vi "Execute.vi"(8 "error in":errorcluster, 11 "Collect Data in":refnum<class "Collect Data.lvclass">) -> (0 "error out":errorcluster, 1 "Next Step?":bool, 2 "MSG":string, 3 "Collect Data out":refnum<class "Collect Data.lvclass">)   [LabVIEW 2015, in "Collect Data.lvclass"]
uses:
  Collect Data.lvclass
  Collect Data.lvclass/Collect Data.ctl
  Reusable/Sequence/STEPS/STEP.lvclass/STEP.ctl
  Reusable/CRDS/Data/Cell/CRDS Cell Data.lvclass/CRDS Cell Data.ctl
  State data/State Data.lvclass
  State data/State Data.lvclass/State Data.ctl
  Reusable/CRDS/Data/Cell/Read extParam.vi
  State data/Write IA.vi
  State data/Write Extinction.vi
  Read # of Obs.vi
  Reusable/Sequence/STEPS/Read First Call.vi
  Read PAS DVR.vi
  Read CRD DVR.vi
  Read Associated Cells.vi
  Read Stored State DVR.vi
  Reusable/Sequence/STEPS/Write First Call.vi
  Reusable/CRDS/Data/Main/Read CellData.vi
  Reusable/Data/Read measTime.vi
  Reusable/PAS/Data/Main/Read CellData.vi
  Reusable/PAS/Data/Cell/Read derived.vi
  Data/cPAS Data.lvclass
  CRDS/Data/cCRDS Data.lvclass
  Reusable/CRDS/Data/Cell/CRDS Cell Data.lvclass
  Reusable/PAS/Data/Cell/PAS Cell Data.lvclass
  <vilib>/Analysis/NI_AALBase.lvlib
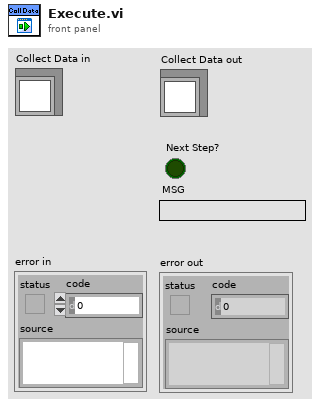
[diagram p1: front panel]
types:
  T1 = typedef "extparam.ctl" = cluster{"Tau":sgl, "Tau0cor":sgl, "ext":sgl, "extCorr":sgl, "stdevTau":sgl, "eTau":sgl, "taucorr":sgl, "Tau0":sgl, "max":sgl}
  T2 = cluster{"f0":sgl, "IA":sgl, "Q":sgl, "max":dbl[], "deltaPhi":dbl, "tau":dbl, "noiseLim":dbl, "ext":dbl}
  T3 = cluster{"Stored State":refnum<class "State Data.lvclass">[], "pointer to data":i32}
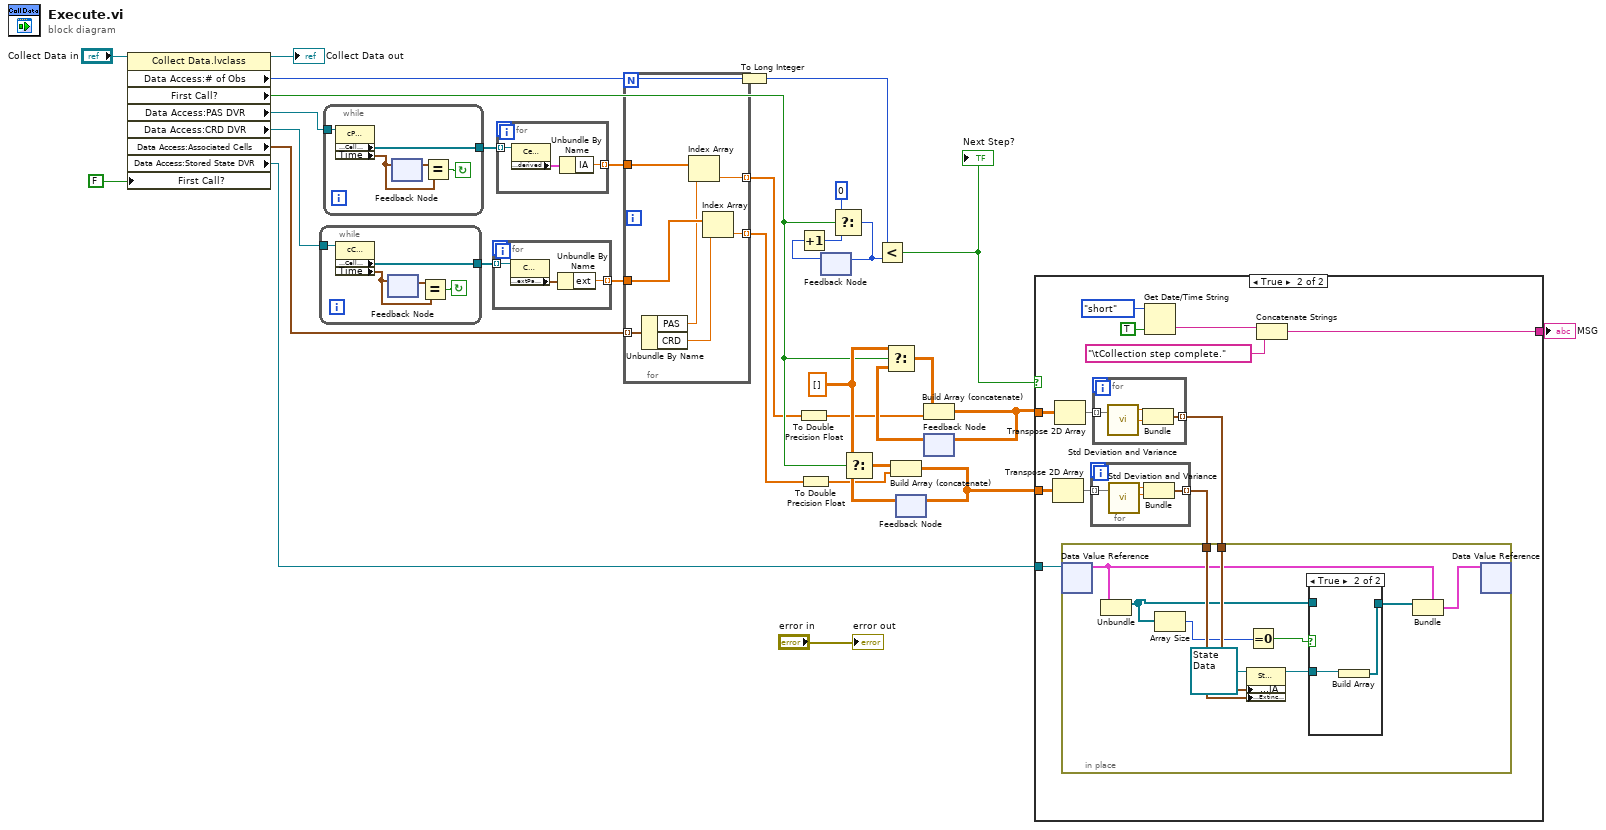
[diagram p0: block diagram]
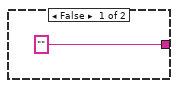
[diagram p2: hidden frame]
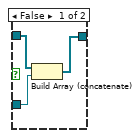
[diagram p3: hidden frame]
diagram:
  w16 = dbl[][] [] ("t")
  n1 = property class="Collect Data.lvclass"(reference="Collect Data in", "First Call?"=FALSE) -> (reference out=→"Collect Data out":refnum<class "Collect Data.lvclass">, "Data Access:# of Obs"=w6:u16, "First Call?"=w7:bool, "Data Access:PAS DVR"=w29:refnum<data-value>, "Data Access:CRD DVR"=w28:refnum<data-value>, "Data Access:Associated Cells"=w11:cluster{"PAS":dbl, "CRD":dbl}[], "Data Access:Stored State DVR"=w19:refnum<data-value>)  [unwired: 1 in, 1 out]
  n2 = while {
    tunnel: w28 -> [w37]
    tunnel: [w36] -> w26
    stop <- w33 continue-if-true
    n3 = property class="cCRDS Data"(reference=w37) -> ("Data Access:Cell Data"=w36:refnum<class "CRDS Cell Data.lvclass">[], "Time"=w35:timestamp)  [unwired: 1 in, 2 out]
    n4 = feedback #1() -> (w34:timestamp)  [unwired: 1 in]
    n5 = feedback-in #1(w35) -> ()
    n6 = Equal?(x=w34, y=w35) -> (x = y?=w33:bool)
  }
  n7 = while {
    tunnel: w29 -> [w42]
    tunnel: [w41] -> w27
    stop <- w40 continue-if-true
    n8 = property class="cPAS Data"(reference=w42) -> ("Data Access:Cell Data"=w41:refnum<class "PAS Cell Data.lvclass">[], "Time"=w38:timestamp)  [unwired: 1 in, 2 out]
    n9 = feedback-in #2(w38) -> ()
    n10 = feedback #2() -> (w39:timestamp)  [unwired: 1 in]
    n11 = Equal?(x=w39, y=w38) -> (x = y?=w40:bool)
  }
  n12 = for {
    tunnel: w26 -> [w45] mode=indexing
    tunnel: [w43] -> w24 mode=indexing
    n13 = property class="CRDS Cell"(reference=w45) -> ("Data Access:extParam"=w44:T1)  [unwired: 1 in, 2 out]
    n14 = Unbundle By Name(w44) -> ("ext"=w43:sgl)
  }
  n15 = for {
    tunnel: w27 -> [w48] mode=indexing
    tunnel: [w46] -> w25 mode=indexing
    n16 = property class="Cell Data"(reference=w48) -> ("Data Access:derived"=w47:T2)  [unwired: 1 in, 2 out]
    n17 = Unbundle By Name(w47) -> ("IA"=w46:sgl)
  }
  n18 = for {
    tunnel: w11 -> [w53] mode=indexing
    tunnel: w25 -> [w55]
    tunnel: w24 -> [w54]
    tunnel: [w50] -> w1 mode=indexing
    tunnel: [w49] -> w4 mode=indexing
    n19 = Unbundle By Name(w53) -> ("PAS"=w52:dbl, "CRD"=w51:dbl)
    n20 = Index Array(array=w55, index=w52) -> (element=w50:sgl)
    n21 = Index Array(array=w54, index=w51) -> (element=w49:sgl)
  }
  n22 = To Long Integer(number=w6) -> (32bit integer=w9:i32)
  n23 = To Double Precision Float(number=w1) -> (double precision float=w2:dbl[])
  n24 = To Double Precision Float(number=w4) -> (double precision float=w3:dbl[])
  n25 = feedback #3() -> (w22:i32)  [unwired: 1 in]
  n26 = Increment(x=w22) -> (x+1=w21:i32)
  n27 = Select(t=0, s=w7, f=w21) -> (s? t:f=w8:i32)
  n28 = feedback-in #3(w8) -> ()
  n29 = Less?(x=w9, y=w8) -> (x < y?=w5:bool)
  "Next Step?" <- w5
  n30 = feedback #4() -> (w14:dbl[][])  [unwired: 1 in]
  n31 = Select(t=w16, s=w7, f=w14) -> (s? t:f=w15:dbl[][])
  n32 = Build Array (concatenate)(w15, w3) -> (w13:dbl[][])
  n33 = feedback-in #4(w13) -> ()
  n34 = feedback #5() -> (w17:dbl[][])  [unwired: 1 in]
  n35 = Select(t=w16, s=w7, f=w17) -> (s? t:f=w20:dbl[][])
  n36 = Build Array (concatenate)(w20, w2) -> (w18:dbl[][])
  n37 = feedback-in #5(w18) -> ()
  n38 = case shown="True" w5 {
    tunnel: w19 -> [_ w68]
    tunnel: w18 -> [_ w67]
    tunnel: w13 -> [_ w66]
    tunnel: ["" w57] -> w12
    frame False {
    }
    frame True {
      n39 = Transpose 2D Array(2D array=w66) -> (transposed array=w64:dbl[][])
      n40 = Transpose 2D Array(2D array=w67) -> (transposed array=w65:dbl[][])
      n41 = for {
        tunnel: w64 -> [w72] mode=indexing
        tunnel: [w69] -> w62 mode=indexing
        n42 = call <vilib>:"Std Deviation and Variance.vi"("X"=w72) -> ("mean"=w71:dbl, "standard deviation"=w70:dbl)  [unwired: 1 in, 1 out]
        n43 = Bundle("mean"=w71, "standard deviation"=w70) -> (w69:cluster{"mean":dbl, "standard deviation":dbl})  [unwired: 1 in]
      }
      n44 = for {
        tunnel: w65 -> [w76] mode=indexing
        tunnel: [w73] -> w63 mode=indexing
        n45 = call <vilib>:"Std Deviation and Variance.vi"("X"=w76) -> ("mean"=w74:dbl, "standard deviation"=w75:dbl)  [unwired: 1 in, 1 out]
        n46 = Bundle("mean"=w74, "standard deviation"=w75) -> (w73:cluster{"mean":dbl, "standard deviation":dbl})  [unwired: 1 in]
      }
      n47 = in-place {
        in-place-border: w63 -> [w86]
        in-place-border: w62 -> [w85]
        n48 = in-place-dvr #6(w68) -> (w84:T3)  [unwired: 1 out]
        n49 = Unbundle(w84) -> ("Stored State"=w77:refnum<class "State Data.lvclass">[])  [unwired: 1 out]
        n50 = Array Size(array=w77) -> (size(s)=w81:i32)
        n51 = property class="State Data"(reference=refnum<class "State Data.lvclass"> refnum, "Data Access:IA"=w86, "Data Access:Extinction"=w85) -> (reference out=w79:refnum<class "State Data.lvclass">)  [unwired: 1 in, 1 out]
        n52 = Equal To 0?(x=w81) -> (x = 0?=w80:bool)
        n53 = case shown="True" w80 {
          tunnel: w79 -> [w89 w91]
          tunnel: [w87 w90] -> w78
          tunnel: w77 -> [w88 _]
          frame False {
            n54 = Build Array (concatenate)(w88, w89) -> (w87:refnum<class "State Data.lvclass">[])
          }
          frame True {
            n55 = Build Array(w91) -> (w90:refnum<class "State Data.lvclass">[])
          }
        }
        n56 = Bundle(cluster=w84, "Stored State"=w78) -> (w83:T3)  [unwired: 1 in]
        n57 = in-place-dvr #6(w83) -> ()  [unwired: 2 out]
      }
      n58 = Get Date/Time String(date format (0)=enum16{"short", "long", "abbreviated"}."short", want seconds? (F)=TRUE) -> (time string=w58:string)  [unwired: 1 in, 1 out]
      n59 = Concatenate Strings(w58, "\tCollection step complete.") -> (w57:string)
    }
  }
  "MSG" <- w12
  "error out" <- "error in"
